vi "Teardown.vi"(8 "Error in":errorcluster, 9 "Unhandled Msgs":refnum<class "Msg.lvclass">[](array[class]), 10 "Lifecycle":T1, 11 "Base Actor in":refnum<class "Base Actor.lvclass">) -> (3 "Base Actor out":refnum<class "Base Actor.lvclass">)   [LabVIEW 2025, in "jettl.lvlib" / "Actor.lvlib" / "Base Actor.lvclass"]
uses:
  Base Actor.lvclass
  Base Actor.lvclass/Base Actor.ctl
  Lifecycle.ctl
  Actor.lvlib
  Msg/Msg.lvclass
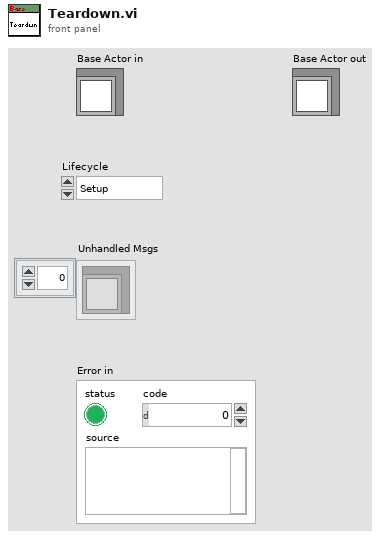
[diagram p1: front panel]
types:
  T1 = typedef "jettl.lvlib/Actor.lvlib/Lifecycle.ctl" = enum16{"Setup", "Teardown"}
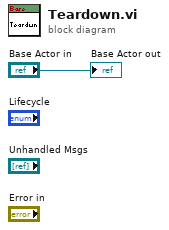
[diagram p0: block diagram]
diagram:
  "Base Actor out" <- "Base Actor in"
